vi "main.vi"() -> ()   [LabVIEW 2020]
uses:
  Controles/Estados_Tablero.ctl
panel:
  in  "Tab Control":enum32{"Tablero Buscaminas", ""}(tab)
  in  "Btn_Inicio_Partida":cluster{"img":u16, " Btn_Inicio":bool}
  out "Mensaje":string
  in  "Tablero":cluster{"img":u16, " Btn_Tablero":bool}[][](array[cluster])
  in  "stop":bool
  in  "Contador":dbl
  # "BUSCAMINAS"
  # "Existen 10 minas!"
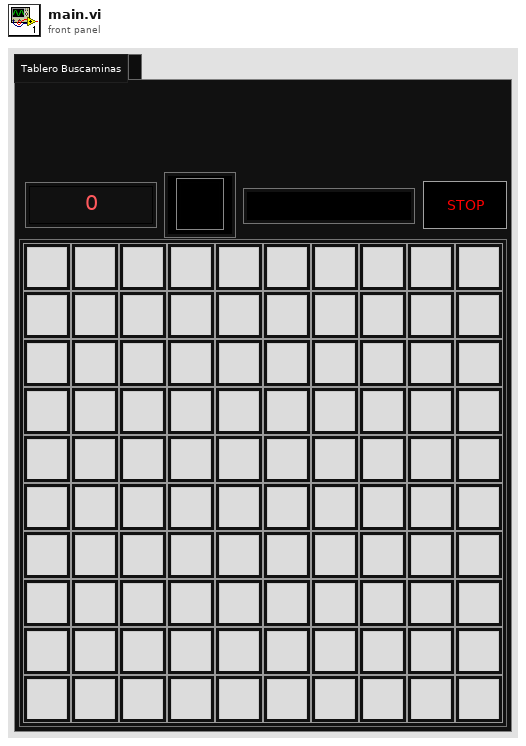
[diagram p1: front panel]
types:
  T1 = typedef "Estados_Tablero.ctl" = enum16{"Inicio", "Jugar", "Ganador", "Perdedor"}
  T2 = cluster{"Posicion":string, "Minas_Alrededor":dbl}[]
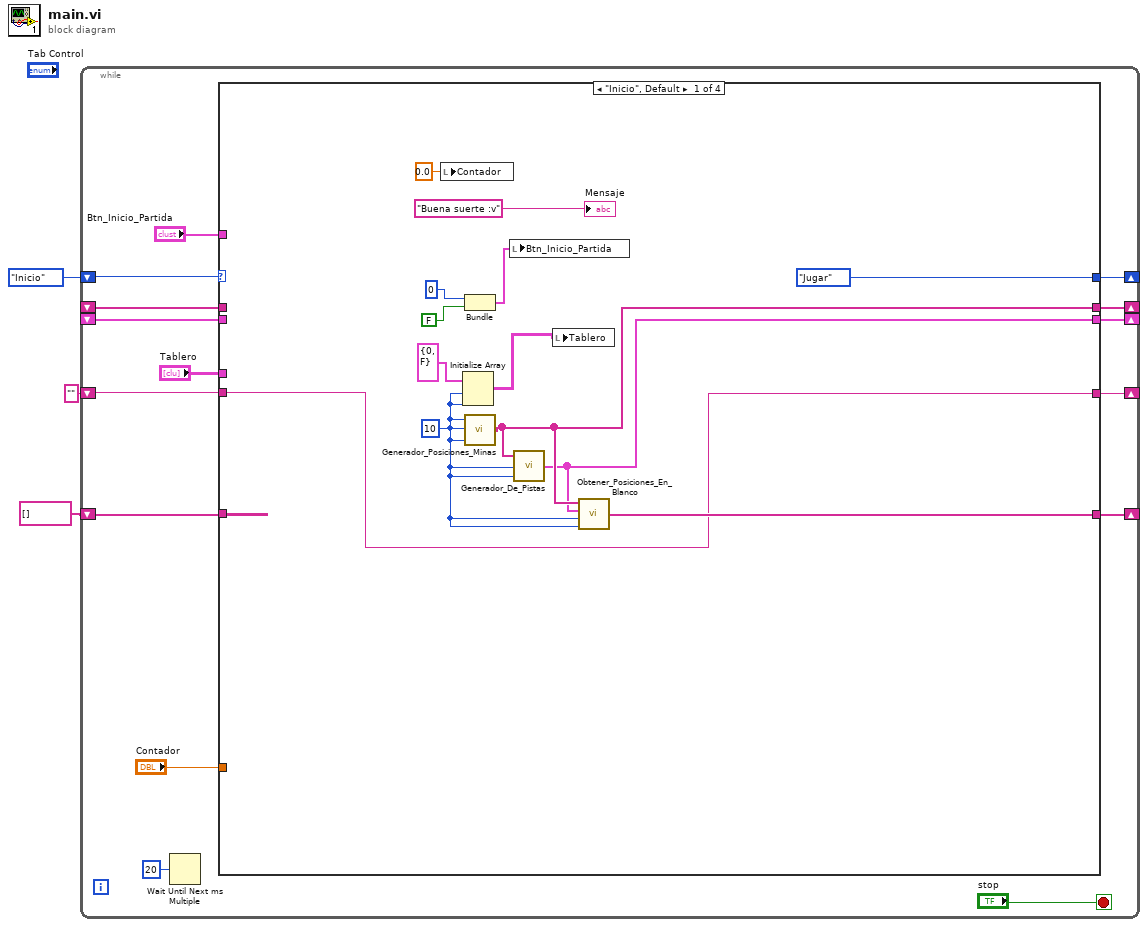
[diagram p0: block diagram]
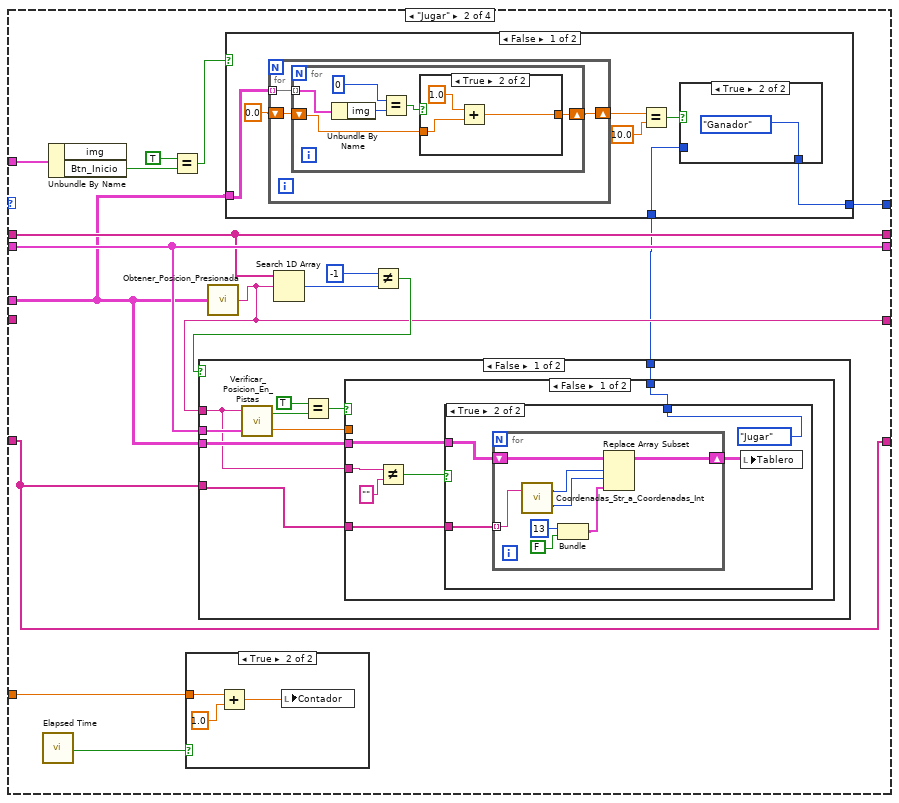
[diagram p2: hidden frame]
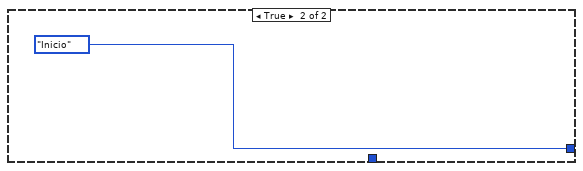
[diagram p6: hidden frame]
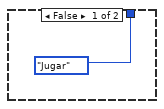
[diagram p7: hidden frame]
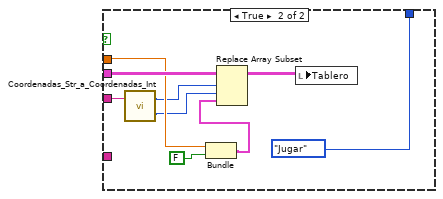
[diagram p8: hidden frame]
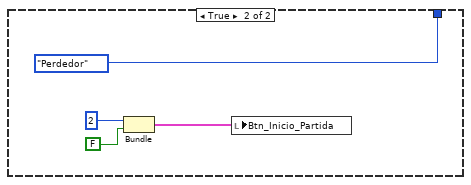
[diagram p9: hidden frame]
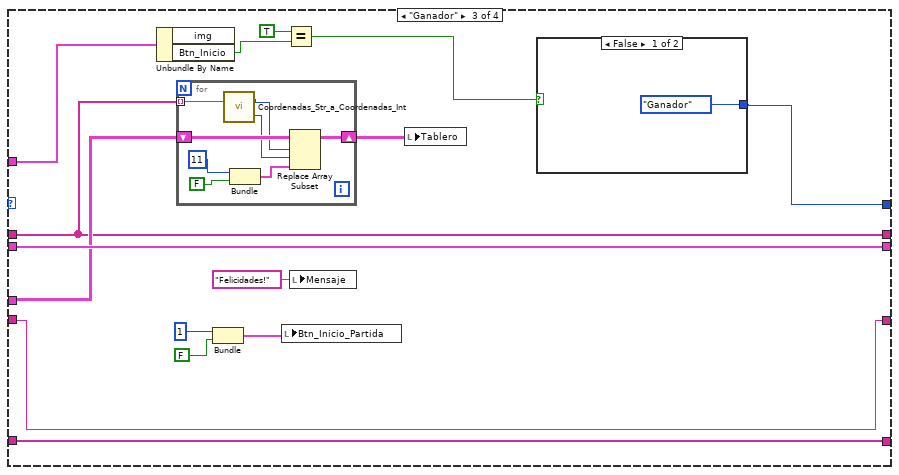
[diagram p10: hidden frame]
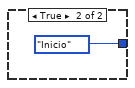
[diagram p11: hidden frame]
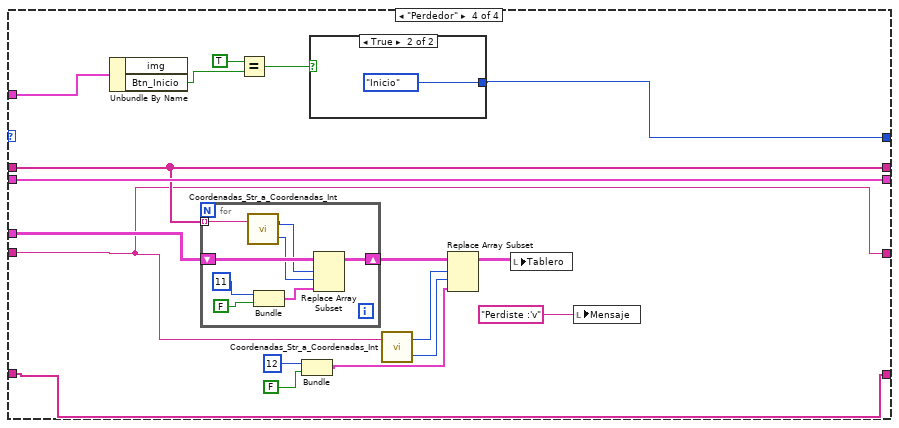
[diagram p12: hidden frame]
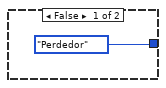
[diagram p13: hidden frame]
diagram:
  n1 = while {
    shift-right: [w16] -> _
    shift-left: Estados_Tablero."Inicio" ("Estados") -> [w17]
    shift-right: [w15] -> _
    shift-left: _ -> [w13]
    shift-right: [w14] -> _
    shift-left: _ -> [w12]
    shift-right: [w11] -> _
    shift-left: string[] [] ("Posiciones_En_Blanco") -> [w10]
    shift-right: [w9] -> _
    shift-left: "" ("Posicion_Presionada") -> [w8]
    stop <- "stop" stop-if-true
    n2 = Wait Until Next ms Multiple(millisecond multiple=u32 20) -> ()  [unwired: 1 out]
    n3 = case shown="\"Inicio\", Default" w17 {
      tunnel: [Estados_Tablero."Jugar" ("Estados") w35 w115 w140] -> w16
      tunnel: [w21 w44 w124 w156] -> w15
      tunnel: [w19 w45 w129 w157] -> w14
      tunnel: w13 -> [_ w44 w124 w156]
      tunnel: w12 -> [_ w45 w129 w157]
      tunnel: "Tablero" -> [_ w34 w126 w155]
      tunnel: [w28 w41 w128 w145] -> w11
      tunnel: w10 -> [_ w41 w128 w145]
      tunnel: [w27 w42 w127 w154] -> w9
      tunnel: w8 -> [w27 _ w127 w154]
      tunnel: "Btn_Inicio_Partida" -> [_ w40 w117 w142]
      tunnel: "Contador" -> [_ w32 _ _]
      frame "Inicio", Default {
        w20 = 10
        n4 = local write "Contador"(0.0 ("Contador")) -> ()
        n5 = Initialize Array(cluster{"img":u16, " Btn_Tablero":bool} {"img"=0, " Btn_Tablero"=FALSE} ("element"), w20, w20) -> (w29:cluster{"img":u16, " Btn_Tablero":bool}[][])
        n6 = Bundle(0, FALSE) -> (w23:cluster{i32, bool})  [unwired: 1 in]
        n7 = call "Generador_Posiciones_Minas.vi"("Num_Columnas"=w20, "Num_Filas"=w20, "Num_Minas"=w20) -> ("Posiciones_Minas"=w21:string[])
        n8 = local write "Btn_Inicio_Partida"(w23) -> ()
        n9 = call "Generador_De_Pistas.vi"("Num_Columnas"=w20, "Num_Filas"=w20, "Posiciones_Minas"=w21) -> ("Pistas"=w19:T2)
        n10 = local write "Tablero"(w29) -> ()
        n11 = call "Obtener_Posiciones_En_Blanco.vi"("Numero_Columnas"=w20, "Numero_Filas"=w20, "Pistas"=w19, "Posiciones_Minas"=w21) -> ("Posiciones_En_Blanco"=w28:string[])
        "Mensaje" <- "Buena suerte :v" ("Mensaje")
      }
      frame "Jugar" {
        n12 = call "Elapsed Time"() -> ("Time has Elapsed"=w33:bool)  [unwired: 12 in, 7 out]
        n13 = Unbundle By Name(w40) -> ("Btn_Inicio"=w39:bool)  [unwired: 1 out]
        n14 = Equal?(x=TRUE, y=w39) -> (x = y?=w37:bool)
        n15 = case shown="True" w33 {
          tunnel: w32 -> [_ w50]
          frame False {
          }
          frame True {
            n16 = Add(x=w50, y=1.0) -> (x+y=w48:dbl)
            n17 = local write "Contador"(w48) -> ()
          }
        }
        n18 = call "Obtener_Posicion_Presionada.vi"("Tablero"=w34) -> ("Posicion_Presionada"=w42:string)
        n19 = Search 1D Array(1D array=w44, element=w42) -> (index of element=w46:i32)  [unwired: 1 in]
        n20 = Not Equal?(x=i16 -1, y=w46) -> (x != y?=w43:bool)
        n21 = case shown="False" w43 {
          tunnel: w45 -> [w82 _]
          tunnel: w42 -> [w76 _]
          tunnel: w34 -> [w77 _]
          tunnel: w41 -> [w75 _]
          tunnel: [w74 Estados_Tablero."Perdedor" ("Estados")] -> w36
          frame False {
            n22 = call "Verificar_Posicion_En_Pistas.vi"("Pistas"=w82, "Posicion"=w76) -> ("Indice_Pista"=w78:dbl, "Es_Una_Pista"=w81:bool)
            n23 = Equal?(x=TRUE, y=w81) -> (x = y?=w79:bool)
            n24 = case shown="False" w79 {
              tunnel: w78 -> [_ w109]
              tunnel: w77 -> [w84 w110]
              tunnel: w76 -> [w88 w107]
              tunnel: w75 -> [w85 _]
              tunnel: [w83 Estados_Tablero."Jugar" ("Estados")] -> w74
              frame False {
                n25 = Not Equal?(x=w88, y="") -> (x != y?=w86:bool)
                n26 = case shown="True" w86 {
                  tunnel: w85 -> [_ w93]
                  tunnel: w84 -> [_ w92]
                  tunnel: [Estados_Tablero."Jugar" ("Estados") Estados_Tablero."Jugar" ("Estados")] -> w83
                  frame False {
                  }
                  frame True {
                    n27 = for {
                      shift-right: [w95] -> w90
                      shift-left: w92 -> [w101]
                      tunnel: w93 -> [w94] mode=indexing
                      n28 = call "Coordenadas_Str_a_Coordenadas_Int.vi"("Coordenadas_Str"=w94) -> ("Columna"=w99:i32, "Fila"=w100:i32)  [unwired: 1 in]
                      n29 = Bundle(13, FALSE) -> (w96:cluster{i32, bool})  [unwired: 1 in]
                      n30 = Replace Array Subset(array=w101, new element=w96, index (row)=w100, index (col)=w99) -> (w95:cluster{"img":u16, " Btn_Tablero":bool}[][])
                    }
                    n31 = local write "Tablero"(w90) -> ()
                  }
                }
              }
              frame True {
                n32 = call "Coordenadas_Str_a_Coordenadas_Int.vi"("Coordenadas_Str"=w107) -> ("Columna"=w105:i32, "Fila"=w106:i32)  [unwired: 1 in]
                n33 = Bundle("Indice_Pista"=w109, FALSE) -> (w104:cluster{"Indice_Pista":dbl, bool})  [unwired: 1 in]
                n34 = Replace Array Subset(array=w110, new element=w104, index (row)=w106, index (col)=w105) -> (w103:cluster{"img":u16, " Btn_Tablero":bool}[][])
                n35 = local write "Tablero"(w103) -> ()
              }
            }
          }
          frame True {
            n36 = Bundle(2, FALSE) -> (w111:cluster{i32, bool})  [unwired: 1 in]
            n37 = local write "Btn_Inicio_Partida"(w111) -> ()
          }
        }
        n38 = case shown="False" w37 {
          tunnel: [w52 Estados_Tablero."Inicio" ("Estados")] -> w35
          tunnel: w36 -> [w51 _]
          tunnel: w34 -> [w57 _]
          frame False {
            n39 = for {
              tunnel: w57 -> [w62] mode=indexing
              shift-right: [w61] -> w55
              shift-left: 0.0 -> [w60]
              n40 = for {
                tunnel: w62 -> [w68] mode=indexing
                shift-right: [w64] -> w61
                shift-left: w60 -> [w63]
                n41 = Unbundle By Name(w68) -> ("img"=w67:u16)
                n42 = Equal?(x=u16 0, y=w67) -> (x = y?=w65:bool)
                n43 = case shown="True" w65 {
                  tunnel: [w69 w71] -> w64
                  tunnel: w63 -> [w69 w70]
                  frame False {
                  }
                  frame True {
                    n44 = Add(x=1.0 ("y"), y=w70) -> (x+y=w71:dbl)
                  }
                }
              }
            }
            n45 = Equal?(x=w55, y=10.0) -> (x = y?=w53:bool)
            n46 = case shown="True" w53 {
              tunnel: [w58 Estados_Tablero."Ganador" ("Estados")] -> w52
              tunnel: w51 -> [w58 _]
              frame False {
              }
              frame True {
              }
            }
          }
          frame True {
          }
        }
      }
      frame "Ganador" {
        n47 = Unbundle By Name(w117) -> ("Btn_Inicio"=w119:bool)  [unwired: 1 out]
        n48 = for {
          shift-right: [w133] -> w125
          shift-left: w126 -> [w139]
          tunnel: w124 -> [w132] mode=indexing
          n49 = call "Coordenadas_Str_a_Coordenadas_Int.vi"("Coordenadas_Str"=w132) -> ("Columna"=w138:i32, "Fila"=w137:i32)  [unwired: 1 in]
          n50 = Bundle(11, FALSE) -> (w134:cluster{i32, bool})  [unwired: 1 in]
          n51 = Replace Array Subset(array=w139, new element=w134, index (row)=w137, index (col)=w138) -> (w133:cluster{"img":u16, " Btn_Tablero":bool}[][])
        }
        n52 = Bundle(1, FALSE) -> (w120:cluster{i32, bool})  [unwired: 1 in]
        n53 = local write "Btn_Inicio_Partida"(w120) -> ()
        n54 = Equal?(x=TRUE, y=w119) -> (x = y?=w116:bool)
        n55 = local write "Mensaje"("Felicidades!" ("Mensaje")) -> ()
        n56 = local write "Tablero"(w125) -> ()
        n57 = case shown="False" w116 {
          tunnel: [Estados_Tablero."Ganador" ("Estados") Estados_Tablero."Inicio" ("Estados")] -> w115
          frame False {
          }
          frame True {
          }
        }
      }
      frame "Perdedor" {
        n58 = Unbundle By Name(w142) -> ("Btn_Inicio"=w144:bool)  [unwired: 1 out]
        n59 = for {
          tunnel: w156 -> [w167] mode=indexing
          shift-right: [w160] -> w151
          shift-left: w155 -> [w166]
          n60 = call "Coordenadas_Str_a_Coordenadas_Int.vi"("Coordenadas_Str"=w167) -> ("Columna"=w165:i32, "Fila"=w164:i32)  [unwired: 1 in]
          n61 = Bundle(11, FALSE) -> (w161:cluster{i32, bool})  [unwired: 1 in]
          n62 = Replace Array Subset(array=w166, new element=w161, index (row)=w164, index (col)=w165) -> (w160:cluster{"img":u16, " Btn_Tablero":bool}[][])
        }
        n63 = Equal?(x=TRUE, y=w144) -> (x = y?=w141:bool)
        n64 = Bundle(12, FALSE) -> (w148:cluster{i32, bool})  [unwired: 1 in]
        n65 = case shown="True" w141 {
          tunnel: [Estados_Tablero."Perdedor" ("Estados") Estados_Tablero."Inicio" ("Estados")] -> w140
          frame False {
          }
          frame True {
          }
        }
        n66 = call "Coordenadas_Str_a_Coordenadas_Int.vi"("Coordenadas_Str"=w154) -> ("Columna"=w149:i32, "Fila"=w150:i32)  [unwired: 1 in]
        n67 = Replace Array Subset(array=w151, new element=w148, index (row)=w150, index (col)=w149) -> (w147:cluster{"img":u16, " Btn_Tablero":bool}[][])
        n68 = local write "Tablero"(w147) -> ()
        n69 = local write "Mensaje"("Perdiste :'v" ("Mensaje")) -> ()
      }
    }
  }
